vi "Is Red Pitaya.vi"(7 "Logic tags":u16[](array[numeric])=[101, 102], 8 "Error In":errorcluster, 10 "Timeout":u32, 11 "connection":refnum<visa-resource-name>) -> (0 "Error Out":errorcluster, 2 "IDN response":u32=1 format="0x%x (%d)", 3 "Red Pitaya":bool, 4 "Error cleared?":bool, 5 "Logic tag out":u16)   [LabVIEW 2015, in "RP Communicator VISA.lvclass"]
uses:
  RP Communicator VISA.lvclass
  <vilib>/Utility/error.llb/Error Cluster From Error Code.vi
  <vilib>/ErrorRing/Error Ring.xnode
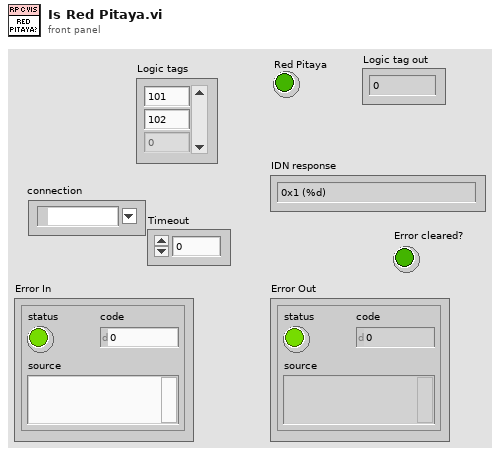
[diagram p1: front panel]
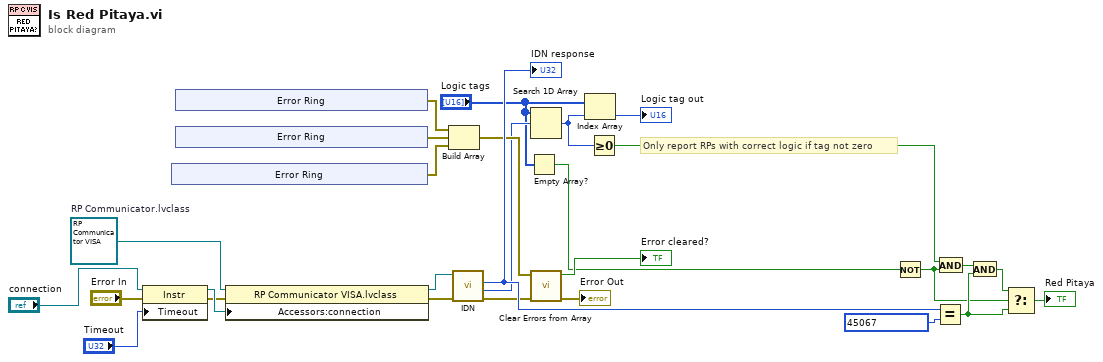
[diagram p0: block diagram]
diagram:
  w28 = refnum<class "RP Communicator VISA.lvclass"> refnum  # RP Communicator.lvclass
  # "Only report RPs with correct logic if tag not zero"
  n1 = property class="Instr"(reference="connection", error in="Error In", "Timeout"="Timeout") -> (reference out=w4:refnum<visa-resource-name>, error out=w2:errorcluster)
  n2 = xnode "Error Ring"() -> ("error out"=w16:errorcluster)
  n3 = xnode "Error Ring"() -> ("error out"=w15:errorcluster)
  n4 = xnode "Error Ring"() -> ("error out"=w17:errorcluster)
  n5 = property class="RP Communicator VISA.lvclass"(reference=w28, error in=w2, "Accessors:connection"=w4) -> (reference out=w27:refnum<class "RP Communicator VISA.lvclass">, error out=w26:errorcluster)
  n6 = Build Array(w15, w17, w16) -> (w14:errorcluster[])
  n7 = call-dynamic "IDN.vi"("error in (no error)"=w26, "RP Communicator in"=w27) -> ("error out"=w19:errorcluster, "Logic tag"=w12:u16, "IDN response"=w23:u32)  [unwired: 6 in, 1 out]
  "IDN response" <- w23
  n8 = Empty Array?(array="Logic tags") -> (empty?=w9:bool)
  n9 = Search 1D Array(1D array="Logic tags", element=w12) -> (index of element=w7:i32)  [unwired: 1 in]
  n10 = call "Clear Errors from Array.vi"("Error In"=w19, "Errors to clear"=w14) -> ("Error Out"=→"Error Out":errorcluster, "specific error cleared?"=→"Error cleared?":bool)  [unwired: 8 in]
  n11 = Index Array(array="Logic tags", index=w7) -> (element=→"Logic tag out":u16)
  n12 = Greater Or Equal To 0?(x=w7) -> (x >= 0?=w6:bool)
  n13 = Not(x=w9) -> (.not. x?=w8:bool)
  n14 = Equal?(x=w23, y=u32 45067 ("IDN response")) -> (x = y?=w21:bool)
  n15 = And(x=w6, y=w8) -> (x .and. y?=w20:bool)
  n16 = And(x=w20, y=w21) -> (x .and. y?=w22:bool)
  n17 = Select(t=w22, s=w8, f=w21) -> (s? t:f=→"Red Pitaya":bool)
